vi "AI Continuous FPGA.vi"() -> ()   [LabVIEW 2019]
uses:
  <vilib>/LabVIEW Targets/FPGA/RIO/BlueMoonOnboardIO/nicrio_cRIO-BlueMoonOnboardAi_VoltageRange.ctl
  <vilib>/LabVIEW Targets/FPGA/RIO/BlueMoonOnboardIO/nicrio_cRIO-BlueMoonOnboardAi_TerminalMod.ctl
  <vilib>/Platform/TimedLoop/XDataNode/timing_clust.ctl
  <vilib>/Platform/TimedLoop/XDataNode/nitl_modes.ctl
  <vilib>/Platform/TimedLoop/XDataNode/wakeup.ctl
  <vilib>/rvi/Emulation/niFpgaGetClockAttributes.vi
  <vilib>/rvi/Emulation/niFpgaSctlEmulationGetInTimedLoop.vi
  <vilib>/rvi/Emulation/niFpgaEmulationReportErrorSimple.vi
  <vilib>/rvi/Emulation/niFpgaCriticalErrorInLSC.vi
  <vilib>/rvi/Emulation/niFpgaProcessEmulError.vi
  <vilib>/rvi/eio/common/nirviEmuTemplateMethod_errors.vi
  <vilib>/rvi/interface/RandomDataEmulation/niFpgaRandomDataHandleErrors.vi
  <vilib>/Platform/TimedLoop/XDataNode/XDataNode.xnode
  <vilib>/eio/EIOMethodNode/EIOMethodNode.xnode
  <vilib>/rvi/DataTransferAndStorage/Container/XNode/niFpgaContainer.xnode
  <vilib>/rvi/interface/RandomDataEmulation/nirviRandomDataFpgaReadWriteTemplate.vi
  <vilib>/Platform/TimedLoop/XDataNode/XDNodeRunTimeDep.lvlib
panel:
  out "Data [i] 2":fxp<+/-,24,5>
  out "Data [i]":fxp<+/-,24,5>
  in  "A?B":bool
  in  "Channel Number [i + 1]":u8
  in  "Terminal Mode [i + 1]":T1=1 items=["DIFF", "RSE"]
  in  "Voltage Range [i + 1]":T2 items=["+/- 10V", "+/- 5V", "+/- 2V", "+/- 1V"]
  in  "Sample time":u32 format="%.0p"
  in  "Start":bool
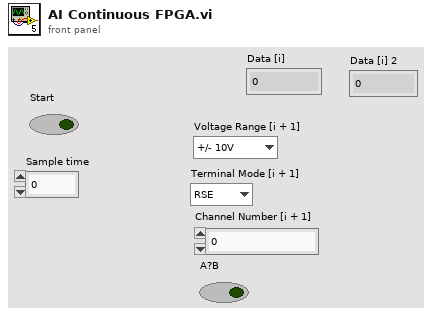
[diagram p1: front panel]
types:
  T1 = typedef "nicrio_cRIO-BlueMoonOnboardAi_TerminalMod.ctl" = u8
  T2 = typedef "nicrio_cRIO-BlueMoonOnboardAi_VoltageRange.ctl" = u8
  T3 = typedef "XDNodeRunTimeDep.lvlib/timing_clust.ctl" = cluster{"Expected End [f-1]":u64, "Actual End [f-1]":u64, "Finished Late? [f-1]":bool, "Expected End [i-1]":u64, "Actual End [i-1]":u64, "Finished Late? [i-1]":bool, "Expected Start [i]":u64, "Actual Start [i]":u64, "Expected Start [f]":u64, "Actual Start [f]":u64, "Source Name":string, "Structure Name":string, "Period":i64, "Deadline":i64, "Offset":i64, "Start":i64, "Priority":i32, "Timeout":i32, "Mode":T4, "Wakeup Reason":T5, "Error":errorcluster, "Source Type":string, "Secondary Source Type":string, "Global End Time":u64, "Global Start Time":u64, "Frame Duration":u64, "Iteration Duration":u64, "Assigned CPU":i32, "I/O Scan Engine Mode":u32}
  T4 = typedef "XDNodeRunTimeDep.lvlib/nitl_modes.ctl" = enum32{"No Change", "Process missed periods, maintain original phase", "Discard missed periods, maintain original phase", "Process missed periods, ignore original phase", "Discard missed periods, ignore original phase"}
  T5 = typedef "XDNodeRunTimeDep.lvlib/wakeup.ctl" = enum32{"Normal", "Aborted", "Asynchronous wakeup", "Timing source error", "Timed loop error", "Timeout"}
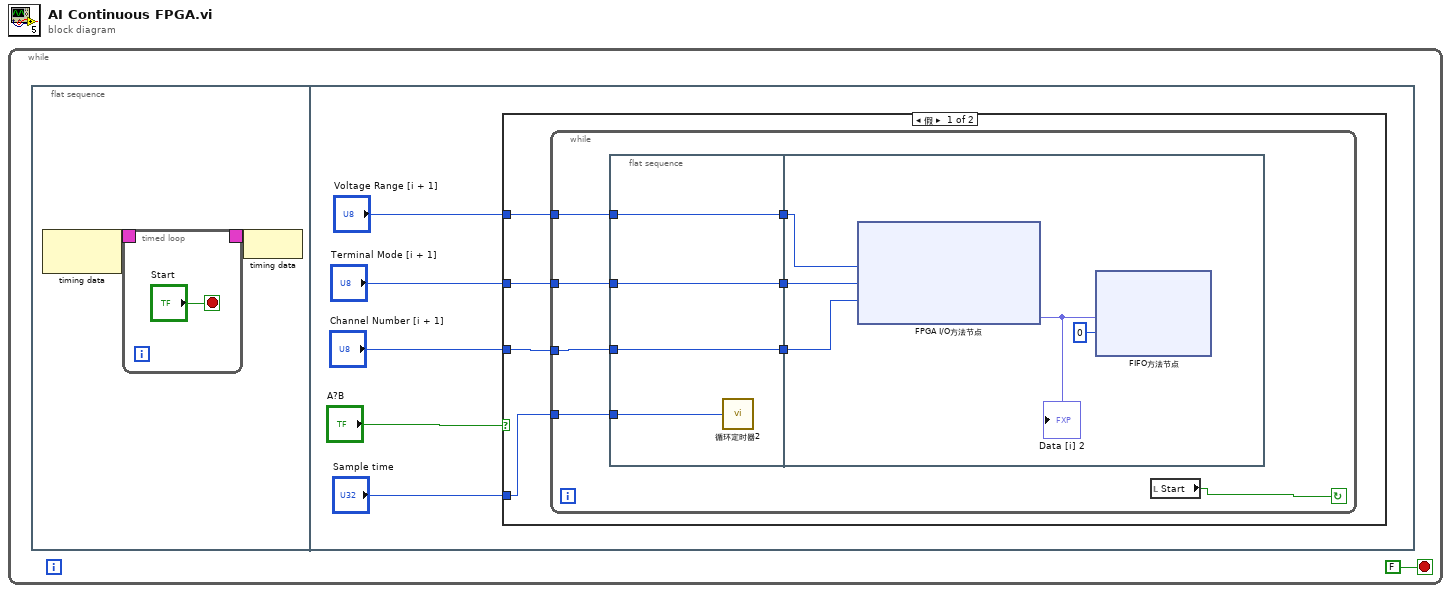
[diagram p0: block diagram]
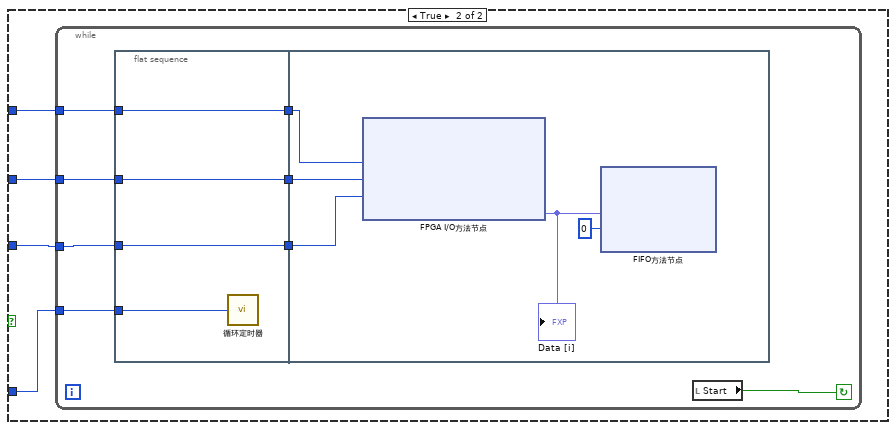
[diagram p2: hidden frame]
diagram:
  n1 = while {
    stop <- FALSE stop-if-true
    n2 = flat-sequence {
      frame #0 {
        n3 = node-c288() -> (w3:T3)  [unwired: 1 in]
        n4 = timed-loop {
          timing: w3 -> [_]
          timing-out: [_] -> w2
          stop <- "Start" stop-if-true
        }
        n5 = node-c288(w2) -> ()
      }
      frame #1 {
        n6 = case shown="假" "A?B" {
          tunnel: "Channel Number [i + 1]" -> [w15 w36]
          tunnel: "Terminal Mode [i + 1]" -> [w16 w37]
          tunnel: "Voltage Range [i + 1]" -> [w17 w38]
          tunnel: "Sample time" -> [w14 w35]
          frame False {
            n7 = while {
              tunnel: w17 -> [w20]
              tunnel: w16 -> [w22]
              tunnel: w15 -> [w24]
              tunnel: w14 -> [w19]
              stop <- w18 continue-if-true
              n8 = flat-sequence {
                tunnel: [w29] -> w25
                tunnel: w24 -> [w29]
                tunnel: [w28] -> w23
                tunnel: w22 -> [w28]
                tunnel: [w27] -> w21
                tunnel: w20 -> [w27]
                tunnel: w19 -> [w26]
                tunnel: w25 -> [w32]
                tunnel: w23 -> [w33]
                tunnel: w21 -> [w34]
                frame #0 {
                  n9 = call "循环定时器2"("Count(uSec)"=w26) -> ()  [unwired: 1 out]
                }
                frame #1 {
                  n10 = xnode "FPGA I/O方法节点"("Voltage Range [i + 1]"=w34, "Terminal Mode [i + 1]"=w33, "Channel Number [i + 1]"=w32) -> ("Data [i]"=w31:fxp<+/-,24,5>)  [unwired: 1 in, 1 out]
                  "Data [i] 2" <- w31
                  n11 = xnode ("FIFO方法节点")("元素"=w31, "超时"=0) -> ()  [unwired: 1 in, 2 out]
                }
              }
              n12 = local read "Start"() -> (w18:bool)
            }
          }
          frame True {
            n13 = while {
              tunnel: w38 -> [w41]
              tunnel: w37 -> [w43]
              tunnel: w36 -> [w45]
              tunnel: w35 -> [w40]
              stop <- w39 continue-if-true
              n14 = flat-sequence {
                tunnel: [w50] -> w46
                tunnel: w45 -> [w50]
                tunnel: [w49] -> w44
                tunnel: w43 -> [w49]
                tunnel: [w48] -> w42
                tunnel: w41 -> [w48]
                tunnel: w40 -> [w47]
                tunnel: w46 -> [w53]
                tunnel: w44 -> [w54]
                tunnel: w42 -> [w55]
                frame #0 {
                  n15 = call "循环定时器"("Count(uSec)"=w47) -> ()  [unwired: 1 out]
                }
                frame #1 {
                  n16 = xnode "FPGA I/O方法节点"("Voltage Range [i + 1]"=w55, "Terminal Mode [i + 1]"=w54, "Channel Number [i + 1]"=w53) -> ("Data [i]"=w52:fxp<+/-,24,5>)  [unwired: 1 in, 1 out]
                  "Data [i]" <- w52
                  n17 = xnode ("FIFO方法节点")("元素"=w52, "超时"=0) -> ()  [unwired: 1 in, 2 out]
                }
              }
              n18 = local read "Start"() -> (w39:bool)
            }
          }
        }
      }
    }
  }
